vi "DynaGlbs.vi"() -> ()   [LabVIEW 2011]
panel:
  in  "GET2217AIns":i32[](array[numeric])=[10376, 9155, 8850, 8545, 8545, 10986, 8850, 8545, -3663, 305, -4579, -3663, -3968, -3663, 2136, 0, 18005, 18005, 16174, 15259, 16479, 16785, 16479, 15564, 305, 305, 305, 305, 305, 305, 305, 305, 5493, 4272, -306, 6714, 5493, 3967, -9996949, 7019, 6104, 5798, 5493, 3052, 7935, 5493, 9460, 3357]
  in  "RBFile Path":path
  in  "Aout ReadS":i32[](array[numeric])=[10376, 9155, 8850, 8545, 8545, 10986, 8850, 8545, -3663, 305, -4579, -3663, -3968, -3663, 2136, 0, 18005, 18005, 16174, 15259, 16479, 16785, 16479, 15564, 305, 305, 305, 305, 305, 305, 305, 305, 5493, 4272, -306, 6714, 5493, 3967, -9996949, 7019, 6104, 5798, 5493, 3052, 7935, 5493, 9460, 3357]
  in  "Valve Read":bool[](array[boolean])=[FALSE, FALSE, FALSE, FALSE, FALSE, FALSE, FALSE, FALSE, FALSE, FALSE, FALSE, FALSE, FALSE, FALSE, FALSE, FALSE, FALSE, FALSE, FALSE, FALSE, FALSE, FALSE, FALSE, FALSE, FALSE, FALSE, FALSE, FALSE, FALSE, FALSE, FALSE, FALSE, FALSE, FALSE, FALSE, FALSE, FALSE, FALSE, FALSE, FALSE, FALSE, FALSE, FALSE, FALSE, FALSE, FALSE, FALSE, FALSE, FALSE, FALSE, FALSE, FALSE, FALSE, FALSE, FALSE, FALSE, FALSE, FALSE, FALSE, FALSE, FALSE, FALSE, FALSE, FALSE, FALSE, FALSE, FALSE, FALSE, FALSE, FALSE, FALSE, FALSE, FALSE, FALSE, FALSE, FALSE, FALSE, FALSE, FALSE, FALSE, FALSE, FALSE, FALSE, FALSE, FALSE, FALSE, FALSE, FALSE]
  in  "Aout Read":dbl[](array[numeric])=[0.0, 0.0, 0.0, 0.0, 0.0, 0.0, 0.0, 0.0, 0.0, 0.0, 0.0, 0.0, 0.0, 0.0, 0.0, 0.0, 0.0, 0.0, 4294967295.0, 0.0, 0.0, 0.0, 0.0, 0.0, 0.0, 0.0, 0.0, 0.0, 4294967295.0, 4294967295.0, 0.0, 0.0, 0.0, 0.0, 0.0, 0.0, 0.0, 0.0, 0.0, 0.0, 0.0, 0.0, 4294967295.0, 4294967295.0, 4294967295.0, 4294967295.0, 4294967295.0, 4294967295.0] format="%.2f"
  in  "EQ Delay":u32=30000
  in  "Serial Init":bool
  in  "N2 Timer":u32
  in  "N2 Cond":bool
  in  "EPS Set":dbl[](array[numeric]) format="%.3f"
  in  "current user":i32
  in  "EPS On":u8[](array[numeric])
  in  "GV/Vac?":bool
  in  "GV/LL?":bool
  in  "Valves rcp":bool[](array[boolean])=[FALSE, FALSE, FALSE, FALSE, FALSE, FALSE, FALSE, FALSE, FALSE, FALSE, FALSE, FALSE, FALSE, FALSE, FALSE, FALSE, FALSE, FALSE, FALSE, FALSE, FALSE, FALSE, FALSE, FALSE, FALSE, FALSE, FALSE, FALSE, FALSE, FALSE, FALSE, FALSE, FALSE, FALSE, FALSE, FALSE, FALSE, FALSE, FALSE, FALSE, FALSE, FALSE, FALSE, FALSE, FALSE, FALSE, FALSE, FALSE, FALSE, FALSE, FALSE, FALSE, FALSE, FALSE, FALSE, FALSE, FALSE, FALSE, FALSE, FALSE, FALSE, FALSE, FALSE, FALSE, FALSE, FALSE, FALSE, FALSE, FALSE, FALSE, FALSE, FALSE, FALSE, FALSE, FALSE, FALSE, FALSE, FALSE, FALSE, FALSE, FALSE, FALSE, FALSE, FALSE, FALSE, FALSE, FALSE, FALSE]
  in  "Program Root":path
  in  "New Layer":bool
  in  "New Dout":bool
  in  "Valves old":bool[](array[boolean])=[FALSE, FALSE, FALSE, FALSE, FALSE, FALSE, FALSE, FALSE, FALSE, FALSE, FALSE, FALSE, FALSE, FALSE, FALSE, FALSE, FALSE, FALSE, FALSE, FALSE, FALSE, FALSE, FALSE, FALSE, FALSE, FALSE, FALSE, FALSE, FALSE, FALSE, FALSE, FALSE, FALSE, FALSE, FALSE, FALSE, FALSE, FALSE, FALSE, FALSE, FALSE, FALSE, FALSE, FALSE, FALSE, FALSE, FALSE, FALSE, FALSE, FALSE, FALSE, FALSE, FALSE, FALSE, FALSE, FALSE, FALSE, FALSE, FALSE, FALSE, FALSE, FALSE, FALSE, FALSE, FALSE, FALSE, FALSE, FALSE, FALSE, FALSE, FALSE, FALSE, FALSE, FALSE, FALSE, FALSE, FALSE, FALSE, FALSE, FALSE, FALSE, FALSE, FALSE, FALSE, FALSE, FALSE, FALSE, FALSE]
  in  "Users":string[](array[string])=["SUPERVISOR", "OPERATOR", "ENGINEER"]
  in  "Passwords":string[](array[string])=["SUPERPOWER", "EMCORE", "SOFTWARE"]
  in  "Done":bool
  in  "Layer count":u8
  in  "Int":bool
  in  "Din":bool[](array[boolean])=[FALSE, FALSE, FALSE, FALSE, FALSE, FALSE, FALSE, FALSE, FALSE, FALSE, FALSE, FALSE, FALSE, FALSE, FALSE, FALSE, FALSE, FALSE, FALSE, FALSE, FALSE, FALSE, FALSE, FALSE, FALSE, FALSE, FALSE, FALSE, FALSE, FALSE, FALSE, FALSE]
  in  "Ain":dbl[](array[numeric])=[0.0, 0.0, 0.0, 0.0, 0.0, 0.0, 0.0, 0.0, 0.0, 0.0, 0.0, 0.0, 0.0, 0.0, 0.0, 0.0, 0.0, 0.0, 0.0, 0.0, 0.0, 0.0, 0.0, 0.0, 0.0, 0.0, 0.0, 0.0, 0.0, 0.0, 0.0, 0.0, 0.0, 0.0, 0.0, 0.0, 0.0, 0.0, 0.0, 0.0, 0.0, 0.0] format="%.2f"
  in  "AOUTS old":dbl[](array[numeric])=[0.0, 0.0, 0.0, 0.0, 0.0, 0.0, 0.0, 0.0, 0.0, 0.0, 0.0, 0.0, 0.0, 0.0, 0.0, 0.0, 0.0, 0.0, 4294967295.0, 0.0, 0.0, 0.0, 0.0, 0.0, 0.0, 0.0, 0.0, 0.0, 4294967295.0, 4294967295.0, 0.0, 0.0, 0.0, 0.0, 0.0, 0.0, 0.0, 0.0, 0.0, 0.0, 0.0, 0.0, 4294967295.0, 4294967295.0, 4294967295.0, 4294967295.0, 4294967295.0, 4294967295.0] format="%.2f"
  in  "Digital mask":bool[](array[boolean])
  in  "States":u8=7
  in  "AInS":i32[](array[numeric])=[10376, 9155, 8850, 8545, 8545, 10986, 8850, 8545, -3663, 305, -4579, -3663, -3968, -3663, 2136, 0, 18005, 18005, 16174, 15259, 16479, 16785, 16479, 15564, 305, 305, 305, 305, 305, 305, 305, 305, 5493, 4272, -306, 6714, 5493, 3967, -9996949, 7019, 6104, 5798, 5493, 3052, 7935, 5493, 9460, 3357]
  in  "New Aout":bool
  in  "Aout Update":bool
  in  "Valves":bool[](array[boolean])=[FALSE, FALSE, FALSE, FALSE, FALSE, FALSE, FALSE, FALSE, FALSE, FALSE, FALSE, FALSE, FALSE, FALSE, FALSE, FALSE, FALSE, FALSE, FALSE, FALSE, FALSE, FALSE, FALSE, FALSE, FALSE, FALSE, FALSE, FALSE, FALSE, FALSE, FALSE, FALSE, FALSE, FALSE, FALSE, FALSE, FALSE, FALSE, FALSE, FALSE, FALSE, FALSE, FALSE, FALSE, FALSE, FALSE, FALSE, FALSE, FALSE, FALSE, FALSE, FALSE, FALSE, FALSE, FALSE, FALSE, FALSE, FALSE, FALSE, FALSE, FALSE, FALSE, FALSE, FALSE, FALSE, FALSE, FALSE, FALSE, FALSE, FALSE, FALSE, FALSE, FALSE, FALSE, FALSE, FALSE, FALSE, FALSE, FALSE, FALSE, FALSE, FALSE, FALSE, FALSE, FALSE, FALSE, FALSE, FALSE]
  in  "AOUTS":dbl[](array[numeric])=[0.0, 0.0, 0.0, 0.0, 0.0, 0.0, 0.0, 0.0, 0.0, 0.0, 0.0, 0.0, 0.0, 0.0, 0.0, 0.0, 0.0, 0.0, 0.0, 0.0, 0.0, 0.0, 0.0, 0.0, 0.0, 0.0, 0.0, 0.0, 0.0, 0.0, 0.0, 0.0, 0.0, 0.0, 0.0, 0.0, 0.0, 0.0, 0.0, 0.0, 0.0, 0.0] format="%.2f"
  # "Security"
  # "Digital I/O"
  # "I/O Control"
  # "Analog I/O"
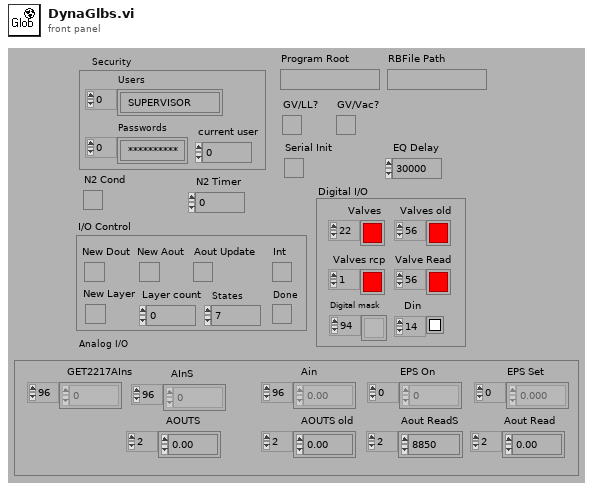
[diagram p1: front panel]
diagram:
